vi "Get google_protobuf_Enum.vi"(8 "error in (no error)":errorcluster, 11 "gRPCid":T1) -> (0 "error out":errorcluster, 2 "package_templatemessage":T2, 3 "gRPCid out":T1)   [LabVIEW 2021, in "ni.measurementlink.measurement.v2.api.lvlib"]
uses:
  ni.measurementlink.measurement.v2.api.lvlib
  google_protobuf_Enum.ctl
  google_protobuf_EnumValue.ctl
  google_protobuf_Option.ctl
  google_protobuf_Any.ctl
  google_protobuf_SourceContext.ctl
  google_protobuf_Syntax.ctl
  <vilib>/gRPC/LabVIEW gRPC Library/Shared/grpcId.ctl
  google_protobuf_Enum_Flat.ctl
  google_protobuf_EnumValue_Flat.ctl
  google_protobuf_Option_Flat.ctl
  google_protobuf_Any_Flat.ctl
  google_protobuf_SourceContext_Flat.ctl
  2ed25e12-861d-4677-8ead-ace2906b2041.vi
  <vilib>/gRPC/LabVIEW gRPC Library/Shared/TranslateGrpcError.vi
  FlatToRichgoogle_protobuf_EnumValue.vi
  FlatToRichgoogle_protobuf_Option.vi
  FlatToRichgoogle_protobuf_SourceContext.vi
  FlatToRichgoogle_protobuf_Any.vi
  <vilib>/gRPC/LabVIEW gRPC Library/Server API/Server/Get Server DLL Path.vi
  <vilib>/Utility/error.llb/Error Cluster From Error Code.vi
  <vilib>/gRPC/LabVIEW gRPC Library/grpc-lvsupport-release.lvlib
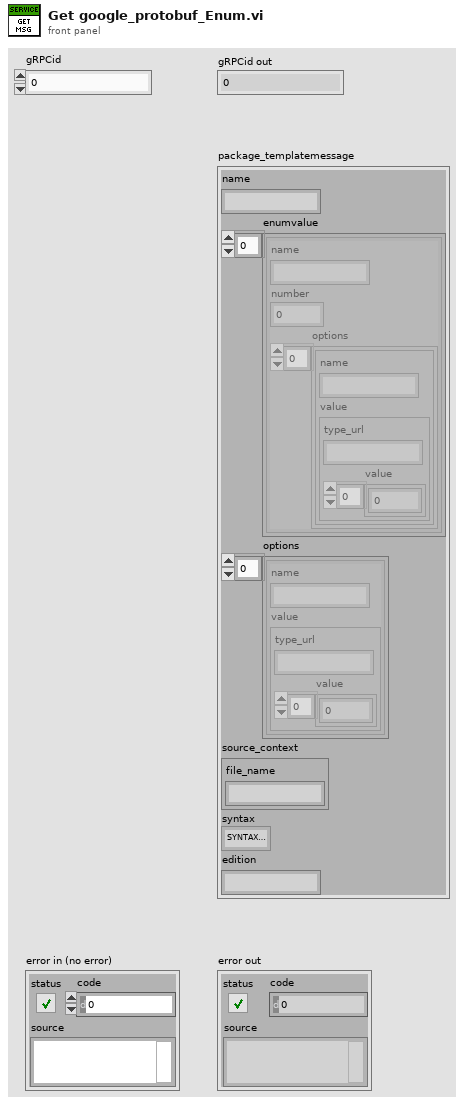
[diagram p1: front panel]
types:
  T1 = typedef "grpc-lvsupport-release.lvlib/grpcId.ctl" = u64
  T2 = typedef "ni.measurementlink.measurement.v2.api.lvlib/google_protobuf_Enum.ctl" = cluster{"name":string, "enumvalue":T3[], "options":T4[], "source_context":T6, "syntax":T7, "edition":string}
  T3 = typedef "ni.measurementlink.measurement.v2.api.lvlib/google_protobuf_EnumValue.ctl" = cluster{"name":string, "number":i32, "options":T4[]}
  T4 = typedef "ni.measurementlink.measurement.v2.api.lvlib/google_protobuf_Option.ctl" = cluster{"name":string, "value":T5}
  T5 = typedef "ni.measurementlink.measurement.v2.api.lvlib/google_protobuf_Any.ctl" = cluster{"type_url":string, "value":u8[]}
  T6 = typedef "ni.measurementlink.measurement.v2.api.lvlib/google_protobuf_SourceContext.ctl" = cluster{"file_name":string}
  T7 = typedef "ni.measurementlink.measurement.v2.api.lvlib/google_protobuf_Syntax.ctl" = enum32{"SYNTAX_PROTO2", "SYNTAX_PROTO3", "SYNTAX_EDITIONS"}
  T8 = typedef "ni.measurementlink.measurement.v2.api.lvlib/google_protobuf_Enum_Flat.ctl" = cluster{"name":string, "enumvalue":T9[], "options":T10[], "source_context":T12, "syntax":T7, "edition":string}
  T9 = typedef "ni.measurementlink.measurement.v2.api.lvlib/google_protobuf_EnumValue_Flat.ctl" = cluster{"name":string, "number":i32, "options":T10[]}
  T10 = typedef "ni.measurementlink.measurement.v2.api.lvlib/google_protobuf_Option_Flat.ctl" = cluster{"name":string, "value":T11}
  T11 = typedef "ni.measurementlink.measurement.v2.api.lvlib/google_protobuf_Any_Flat.ctl" = cluster{"type_url":string, "value":u8[]}
  T12 = typedef "ni.measurementlink.measurement.v2.api.lvlib/google_protobuf_SourceContext_Flat.ctl" = cluster{"file_name":string}
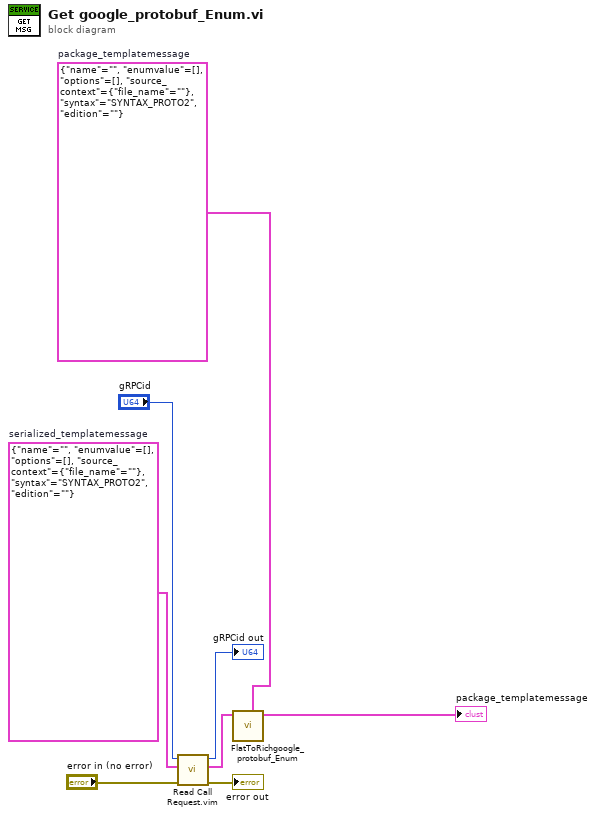
[diagram p0: block diagram]
diagram:
  w6 = T8 {"name"="", "enumvalue"=[], "options"=[], "source_context"={"file_name"=""}, "syntax"=enum."SYNTAX_PROTO2", "edition"=""}  # serialized_templatemessage
  w5 = T2 {"name"="", "enumvalue"=[], "options"=[], "source_context"={"file_name"=""}, "syntax"=enum."SYNTAX_PROTO2", "edition"=""}  # package_templatemessage
  n1 = call "Read Call Request.vim"("error in"="error in (no error)", "Request Type"=w6, "gRPCid in"="gRPCid") -> ("error out"=→"error out":errorcluster, "Request Data"=w4:T8, "gRPCid out"=→"gRPCid out":T1)  [unwired: 6 in]
  n2 = call "FlatToRichgoogle_protobuf_Enum.vi"("OutputClusterType"=w5, "InputCluster"=w4) -> ("OutputCluster"=→"package_templatemessage":T2)  [unwired: 9 in]
